vi "cRIO_Fsensor_testVI.vi"() -> ()   [LabVIEW 2019]
uses:
  <vilib>/Platform/TimedLoop/XDataNode/timing_clust.ctl
  <vilib>/Platform/TimedLoop/XDataNode/nitl_modes.ctl
  <vilib>/Platform/TimedLoop/XDataNode/wakeup.ctl
  <vilib>/Analysis/baseanly.llb/Mean (DBL).vi
  <vilib>/platform/TimedLoop/XDataNode/XDataNode.xnode
  <vilib>/Analysis/NI_AALBase.lvlib
  <vilib>/Platform/TimedLoop/XDataNode/XDNodeRunTimeDep.lvlib
panel:
  out "Raw voltages":dbl[](array[numeric])
  out "F 2":dbl[](array[numeric])
  out "Torques (Nm)":T1(graph)
  out "Forces (N)":T1(graph)
  out "F":dbl[](array[numeric])
  in  "Ftrans":bool=TRUE
  out "TransF":dbl[](array[numeric])
  in  "d_{1}_{2} (mm)":dbl[](array[numeric])=[10.0, 0.0, 0.0]
  in  "Manual force":bool
  in  "Manual forces\n(mouse frame)":dbl[](array[numeric])=[0.0, 0.0, 0.0, 0.0, 0.0, 0.0]
  out "Mouse forces":dbl[](array[numeric])
  in  "Measure Fsensor \nV offset":bool
  out "Sensor V offset":dbl[](array[numeric])
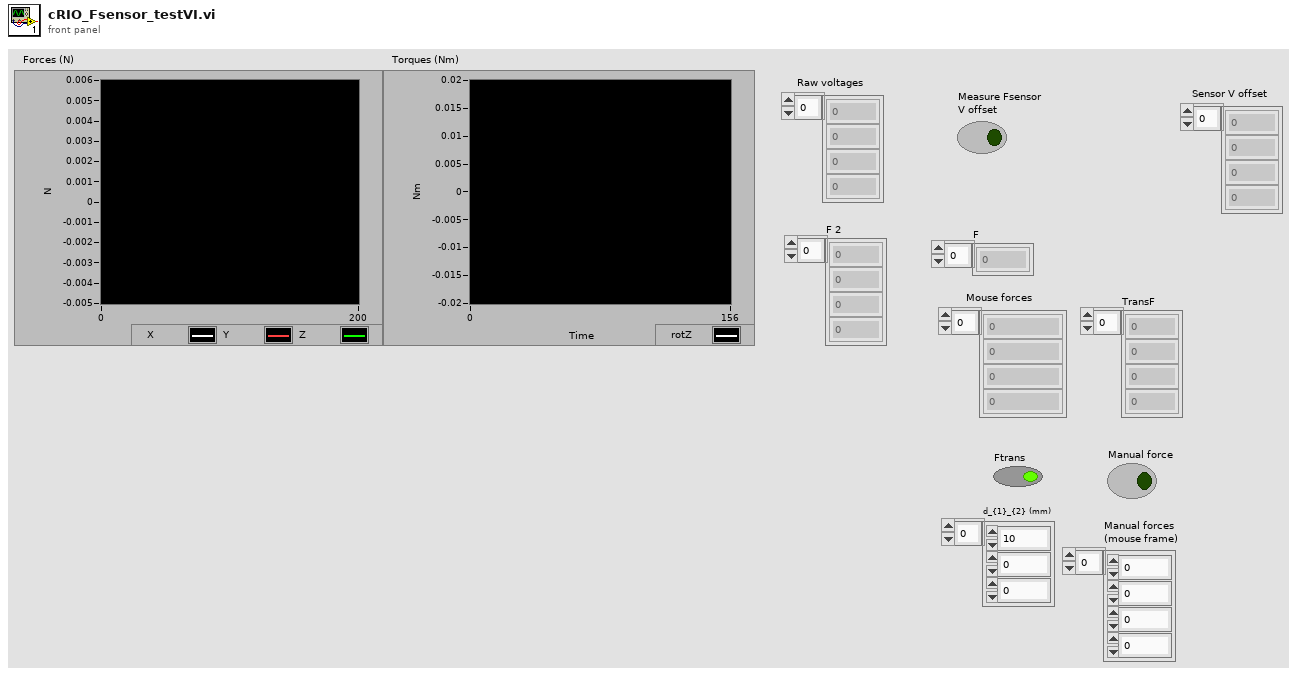
[diagram p1: front panel]
types:
  T1 = cluster{"F[0]":dbl, "F[1]":dbl, "F[2]":dbl, "F[3]":dbl, "F[4]":dbl, "F[5]":dbl, "F[6]":dbl, "F[7]":dbl, "F[8]":dbl}
  T2 = typedef "XDNodeRunTimeDep.lvlib/timing_clust.ctl" = cluster{"Expected End [f-1]":u64, "Actual End [f-1]":u64, "Finished Late? [f-1]":bool, "Expected End [i-1]":u64, "Actual End [i-1]":u64, "Finished Late? [i-1]":bool, "Expected Start [i]":u64, "Actual Start [i]":u64, "Expected Start [f]":u64, "Actual Start [f]":u64, "Source Name":string, "Structure Name":string, "Period":i64, "Deadline":i64, "Offset":i64, "Start":i64, "Priority":i32, "Timeout":i32, "Mode":T3, "Wakeup Reason":T4, "Error":errorcluster, "Source Type":string, "Secondary Source Type":string, "Global End Time":u64, "Global Start Time":u64, "Frame Duration":u64, "Iteration Duration":u64, "Assigned CPU":i32, "I/O Scan Engine Mode":u32}
  T3 = typedef "XDNodeRunTimeDep.lvlib/nitl_modes.ctl" = enum32{"No Change", "Process missed periods, maintain original phase", "Discard missed periods, maintain original phase", "Process missed periods, ignore original phase", "Discard missed periods, ignore original phase"}
  T4 = typedef "XDNodeRunTimeDep.lvlib/wakeup.ctl" = enum32{"Normal", "Aborted", "Asynchronous wakeup", "Timing source error", "Timed loop error", "Timeout"}
  T5 = cluster{"[0]":dbl, "[1]":dbl, "[2]":dbl, "[3]":dbl, "[4]":dbl, "[5]":dbl, "[6]":dbl, "[7]":dbl, "[8]":dbl}
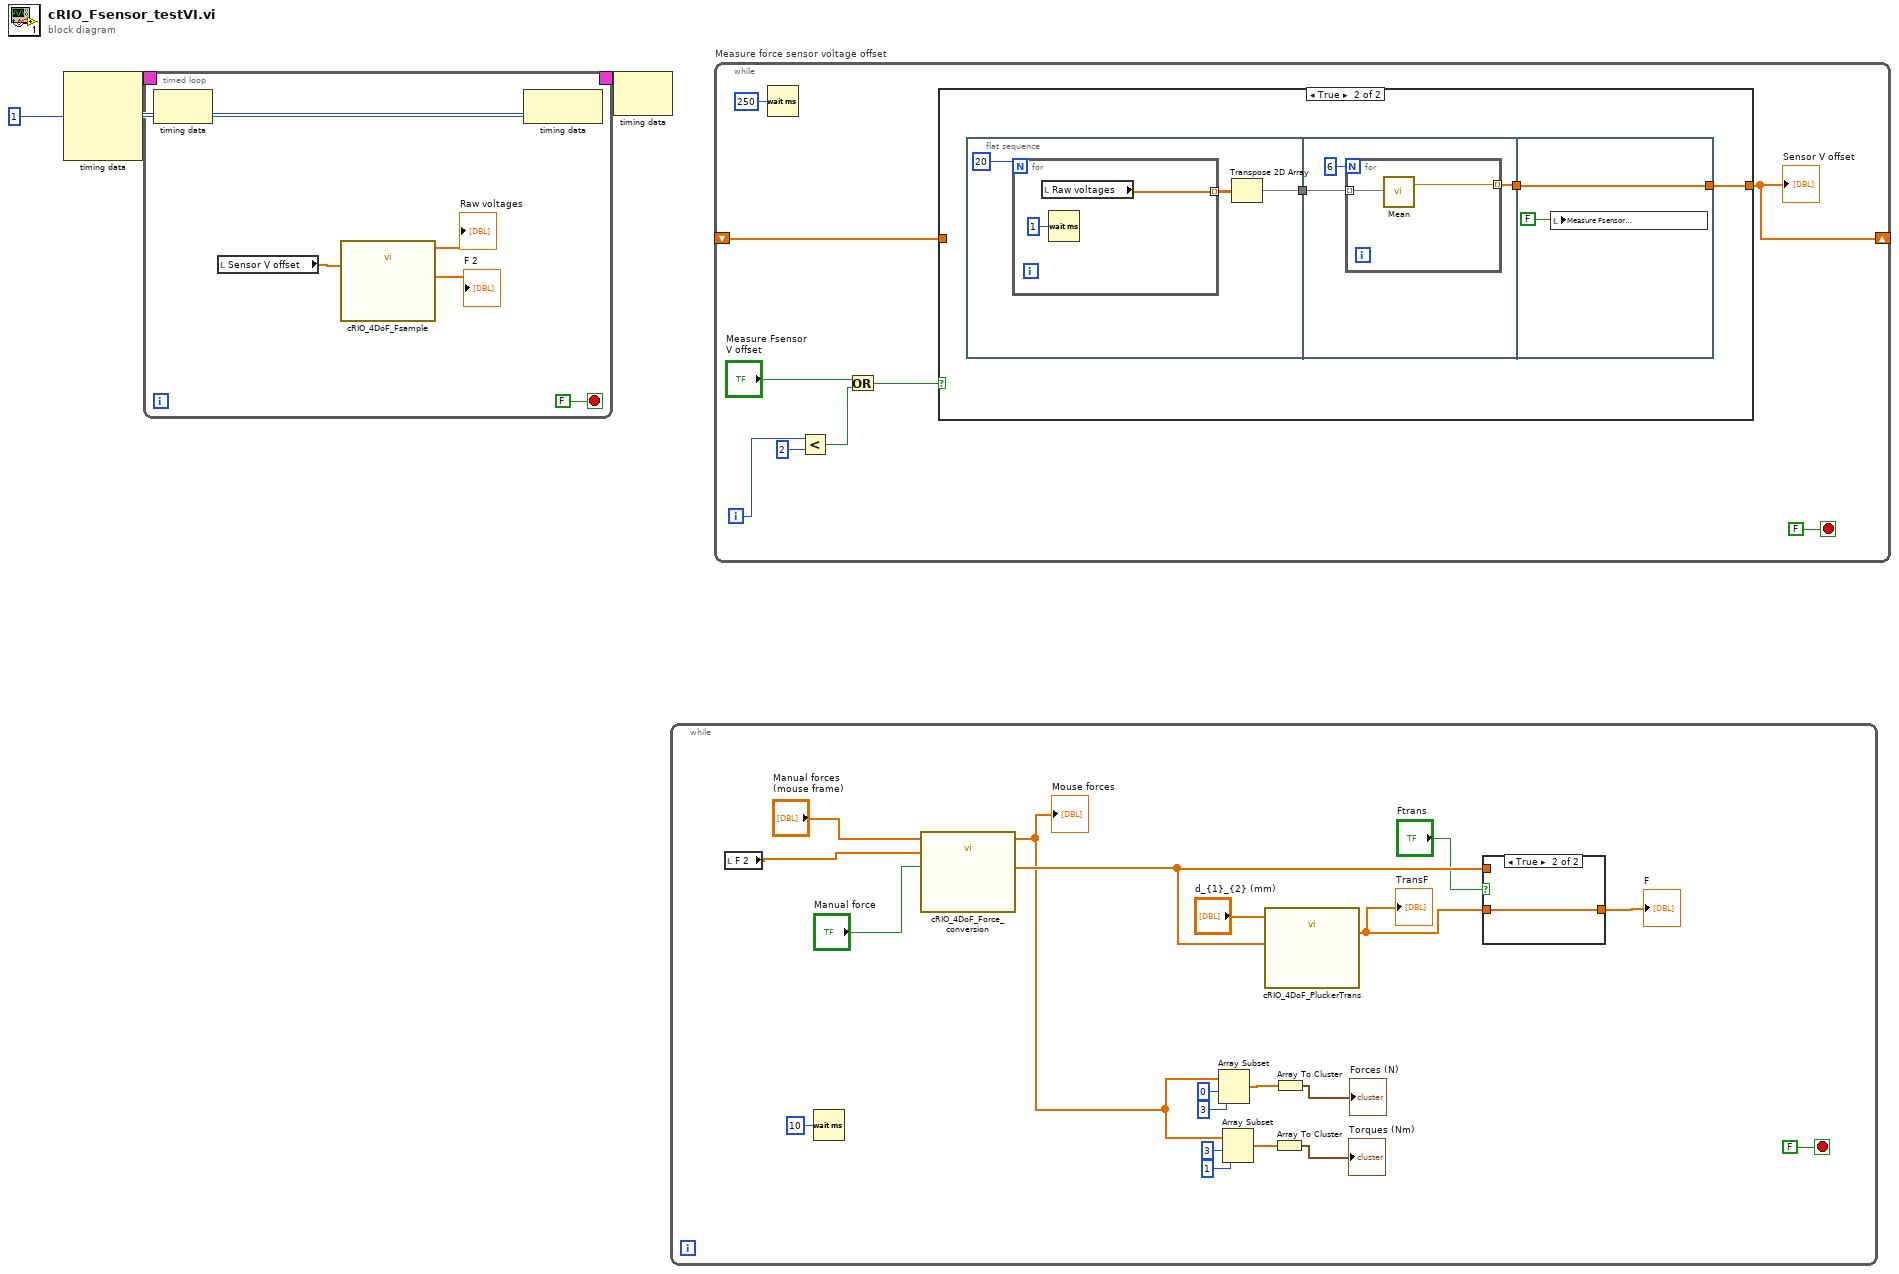
[diagram p0: block diagram]
diagram:
  n1 = node-c288(i64 1 ("Period")) -> (w3:T2)  [unwired: 3 in]
  n2 = timed-loop {
    timing: w3 -> [_]
    timing-out: [_] -> w2
    stop <- FALSE stop-if-true
    n3 = node-c288() -> ()  [unwired: 1 in, 1 out]
    n4 = local read "Sensor V offset"() -> (w7:dbl[])
    n5 = call "cRIO_4DoF_Fsample.vi"("Sensor V offset"=w7) -> ("F"=→"F 2":dbl[], "Array"=→"Raw voltages":dbl[])  [unwired: 9 in]
    n6 = node-c288() -> ()  [unwired: 1 in, 1 out]
  }
  n7 = node-c288(w2) -> ()  [unwired: 1 out]
  n8 = while {
    stop <- FALSE stop-if-true
    n9 = local read "F 2"() -> (w11:dbl[])
    n10 = Wait (ms)(milliseconds to wait=u32 10) -> ()  [unwired: 1 out]
    n11 = call "cRIO_4DoF_Force_conversion.vi"("Manual force"="Manual force", "F_measured"=w11, "Manual forces in"="Manual forces\n(mouse frame)") -> ("Force control"=w24:dbl[], "F_mouse"=w12:dbl[])  [unwired: 7 in]
    "Mouse forces" <- w12
    n12 = Array Subset(array=w12, index=0, length=3) -> (w20:dbl[])
    n13 = Array Subset(array=w12, index=3, length=1) -> (w15:dbl[])
    n14 = call "cRIO_4DoF_PluckerTrans.vi"("Force control"=w24, "d_{1}_{2} (mm)"="d_{1}_{2} (mm)") -> ("TransF"=w25:dbl[])  [unwired: 9 in]
    "TransF" <- w25
    n15 = Array To Cluster(array=w15) -> (cluster=→"Torques (Nm)":T5)
    n16 = Array To Cluster(array=w20) -> (cluster=→"Forces (N)":T5)
    n17 = case shown="True" "Ftrans" {
      tunnel: w25 -> [_ w30]
      tunnel: [w29 w30] -> w21
      tunnel: w24 -> [w29 _]
      frame False {
      }
      frame True {
      }
    }
    "F" <- w21
  }
  n18 = while "Measure force sensor voltage offset" {
    shift-right: [w39] -> _
    shift-left: _ -> [w38]
    i -> [w35]
    stop <- FALSE stop-if-true
    n19 = Wait (ms)(milliseconds to wait=u32 250) -> ()  [unwired: 1 out]
    n20 = Less?(x=w35, y=2) -> (x < y?=w33:bool)
    n21 = Or(x="Measure Fsensor \nV offset", y=w33) -> (x .or. y?=w32:bool)
    n22 = case shown="True" w32 {
      tunnel: [w40 w42] -> w39
      tunnel: w38 -> [w40 _]
      frame False {
      }
      frame True {
        n23 = flat-sequence {
          tunnel: [w44] -> w43
          tunnel: w43 -> [w50]
          tunnel: [w49] -> w41
          tunnel: [w55] -> w42
          tunnel: w41 -> [w55]
          frame #0 {
            n24 = for {
              N: 20 -> [_]
              tunnel: [w48] -> w45 mode=indexing
              n25 = local read "Raw voltages"() -> (w48:dbl[])
              n26 = Wait (ms)(milliseconds to wait=u32 1) -> ()  [unwired: 1 out]
            }
            n27 = Transpose 2D Array(2D array=w45) -> (transposed array=w44:dbl[][])
          }
          frame #1 {
            n28 = for {
              N: 6 -> [_]
              tunnel: w50 -> [w53] mode=indexing
              tunnel: [w52] -> w49 mode=indexing
              n29 = call-poly <vilib>:"Mean.vi"("X"=w53) -> ("mean"=w52:dbl)  [unwired: 1 out]
            }
          }
          frame #2 {
            n30 = local write "Measure Fsensor \nV offset"(FALSE ("DAQ V offset")) -> ()
          }
        }
      }
    }
    "Sensor V offset" <- w39
  }
